vi "GUI Waveform Update.vi"(7 "Destroy notifier (False)":bool, 8 "error in":errorcluster, 11 "sequence item":T1) -> (0 "error out":errorcluster)   [LabVIEW 2018]
doc: "This VI will sends new record notification to the Waveform viewer. Use this whenever you want to update data in the waveform viewer. Call it with parameter 'destroy' somewhere at the application exit to destroy the notifier used for signalisation to the Waveform viewer panel."
uses:
  Meas Sequence Item.ctl
  Meas Sampling Configuration.ctl
  adc/ADC Trig Config.ctl
  adc/ADC Trig Mode Source.ctl
  adc/ADC Trig Coupling.ctl
  adc/ADC Trig Slope.ctl
  processing/QWTB/Meas Proc QWTB Algorithm Parameter Data.ctl
  GUI Waveform Info.ctl
  varilib/varilib.lvlib
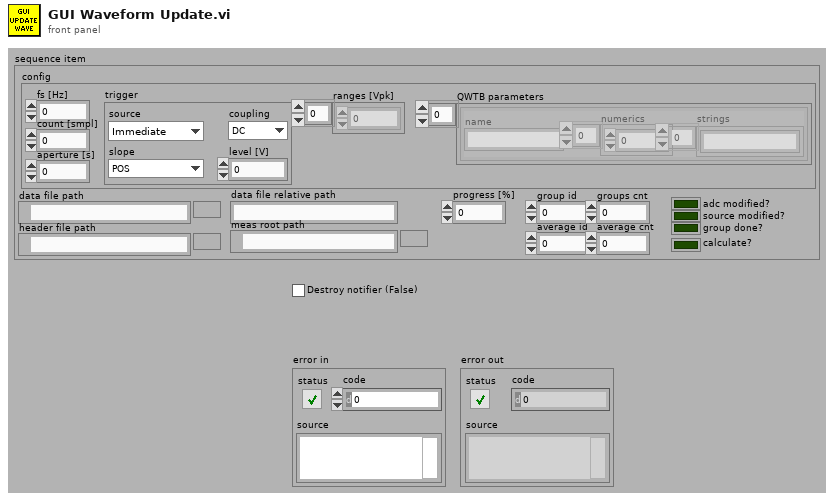
[diagram p1: front panel]
types:
  T1 = typedef "Meas Sequence Item.ctl" = cluster{"config":T2, "data file path":path, "header file path":path, "group id":i32, "average id":i32, "group done?":bool, "adc modified?":bool, "source modified?":bool, "progress [%]":dbl, "groups cnt":i32, "average cnt":i32, "data file relative path":string, "meas root path":path, "calculate?":bool}
  T2 = typedef "Meas Sampling Configuration.ctl" = cluster{"fs [Hz]":dbl, "count [smpl]":i64, "aperture [s]":dbl, "trigger":T3, "ranges [Vpk]":dbl[], "QWTB parameters":T7[]}
  T3 = typedef "ADC Trig Config.ctl" = cluster{"source":T4, "level [V]":dbl, "coupling":T5, "slope":T6}
  T4 = typedef "ADC Trig Mode Source.ctl" = enum16{"Immediate", "External", "Level"}
  T5 = typedef "ADC Trig Coupling.ctl" = enum16{"DC", "AC"}
  T6 = typedef "ADC Trig Slope.ctl" = enum16{"POS", "NEG"}
  T7 = typedef "Meas Proc QWTB Algorithm Parameter Data.ctl" = cluster{"name":string, "numerics":dbl[], "strings":string[]}
  T8 = typedef "GUI Waveform Info.ctl" = cluster{"header path":path, "group id":i32, "average id":i32, "Time Stamp":timestamp, "max samples":i64, "first sample":i64, "first smpl [%]":dbl, "kill viewer":bool}
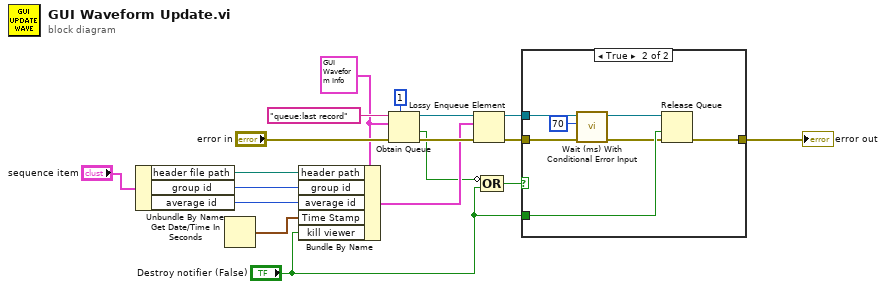
[diagram p0: block diagram]
diagram:
  w10 = T8 {"header path"=path "", "group id"=0, "average id"=0, "Time Stamp"=timestamp(0 s since 1904-01-01), "max samples"=0, "first sample"=0, "first smpl [%]"=0.0, "kill viewer"=FALSE} ("record info")
  n1 = Unbundle By Name("sequence item") -> ("header file path"=w4:path, "group id"=w3:i32, "average id"=w2:i32)
  n2 = Get Date/Time In Seconds() -> (seconds since 1Jan1904=w8:timestamp)
  n3 = Bundle By Name(cluster=w10, "header path"=w4, "group id"=w3, "average id"=w2, "Time Stamp"=w8, "kill viewer"="Destroy notifier (False)") -> (w9:T8)
  n4 = Obtain Queue(max queue size (-1, unlimited)=1, name (unnamed)="queue:last record", element data type=w10, error in (no error)="error in") -> (queue out=w14:refnum<queue>, created new?=w6:bool, error out=w15:errorcluster)  [unwired: 1 in]
  n5 = Lossy Enqueue Element(queue=w14, element=w9, error in (no error)=w15) -> (queue out=w12:refnum<queue>, error out=w13:errorcluster)  [unwired: 2 out]
  n6 = Compound Arithmetic op=OR(invert w6, "Destroy notifier (False)") -> (w7:bool)
  n7 = case shown="True" w7 {
    tunnel: w13 -> [w19 w25]
    tunnel: w12 -> [_ w24]
    tunnel: [w19 w23] -> w11
    tunnel: "Destroy notifier (False)" -> [_ w22]
    frame False {
    }
    frame True {
      n8 = call "Wait (ms) With Conditional Error Input.vi"("error in (no error)"=w25, "milliseconds to wait"=u32 70) -> ("error out"=w21:errorcluster)  [unwired: 8 in, 1 out]
      n9 = Release Queue(queue=w24, force destroy? (F)=w22, error in (no error)=w21) -> (error out=w23:errorcluster)  [unwired: 2 out]
    }
  }
  "error out" <- w11
